vi "Calc_Extention.vi"(8 "Center State at T":T1, 9 "Initial Anchor Position":dbl[][](array[numeric]), 11 "Particle Posi":dbl[][](array[numeric])) -> (0 "Center State at T 2":T1, 3 "Extention":dbl[][](array[numeric]))   [LabVIEW 2020]
uses:
  <vilib>/Analysis/baseanly.llb/Mean (DBL).vi
  <vilib>/Analysis/NI_AALBase.lvlib
panel:
  out "Anchor Posi at T":dbl[][](array[numeric])
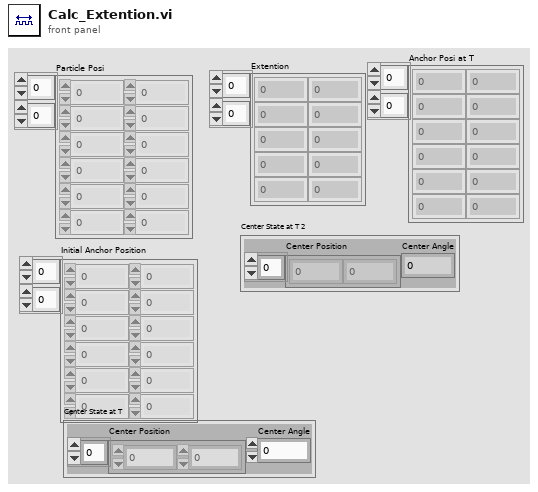
[diagram p1: front panel]
types:
  T1 = cluster{"Center Position":dbl[], "Center Angle":dbl}
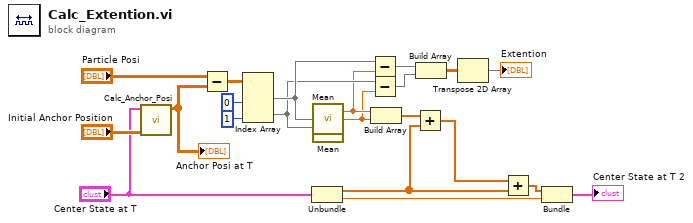
[diagram p0: block diagram]
diagram:
  n1 = call "Calc_Anchor_Posi.vi"("Initial Anchor Position"="Initial Anchor Position", "Center State at T"="Center State at T") -> ("Anchor Posi at T"=w8:dbl[][])  [unwired: 9 in]
  "Anchor Posi at T" <- w8
  n2 = Subtract(x="Particle Posi", y=w8) -> (x-y=w11:dbl[][])
  n3 = Index Array(array=w11, index (col) #1=0 ("disabled index (col)"), index (col) #2=1 ("index (col)")) -> (element #1=w18:dbl[], element #2=w17:dbl[])  [unwired: 2 in]
  n4 = Unbundle("Center State at T") -> ("Center Position"=w3:dbl[], "Center Angle"=w6:dbl)
  n5 = call-poly <vilib>:"Mean.vi"("X"=w18) -> ("mean"=w13:dbl)  [unwired: 1 out]
  n6 = call-poly <vilib>:"Mean.vi"("X"=w17) -> ("mean"=w12:dbl)  [unwired: 1 out]
  n7 = Subtract(x=w18, y=w13) -> (x-y=w16:dbl[])
  n8 = Subtract(x=w17, y=w12) -> (x-y=w15:dbl[])
  n9 = Build Array(w13, w12) -> (w5:dbl[])
  n10 = Add(x=w5, y=w3) -> (x+y=w2:dbl[])
  n11 = Build Array(w16, w15) -> (w14:dbl[][])
  n12 = Transpose 2D Array(2D array=w14) -> (transposed array=→"Extention":dbl[][])
  n13 = Add(x=w2, y=w3) -> (x+y=w1:dbl[])
  n14 = Bundle(w1, "Center Angle"=w6) -> (→"Center State at T 2":cluster{dbl[], "Center Angle":dbl})  [unwired: 1 in]
